vi "Chassis Speed Data.vi"() -> ()   [LabVIEW 2011]
panel:
  in  "Chassis Direction":i16
  in  "Chassis Speed":dbl
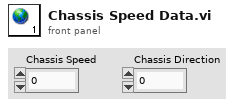
[diagram p1: front panel]
diagram:
